vi "consecutive_false.vi"(10 "bool":bool) -> (2 "sum":u8)   [LabVIEW 2018]
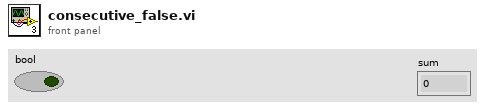
[diagram p1: front panel]
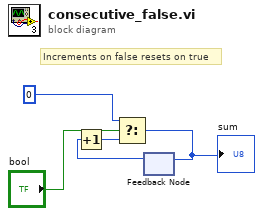
[diagram p0: block diagram]
diagram:
  # "Increments on false resets on true"
  n1 = feedback #1() -> (w3:u8)  [unwired: 1 in]
  n2 = Increment(x=w3) -> (x+1=w2:u8)
  n3 = Select(t=u8 0, s="bool", f=w2) -> (s? t:f=w4:u8)
  "sum" <- w4
  n4 = feedback-in #1(w4) -> ()
